vi "Child_2 - Config - RD WR.vi"(8 "Error In":errorcluster, 9 "Create a New Config File?":bool, 11 "In Cluster":T1={"Relative Array of paths"=["API", "Cfg", "Common", "Data", "Data\\Database_Script", "Data\\FW", "Data\\PIC", "Data\\DBC", "Data\\SSL_Certificates", "Debug", "Deployment", "Documentation", "Driver", "SEQ", "SEQ\\PreUUT\\Control", "SEQ\\PreUUT\\Module", "SEQ\\PreUUT\\Scanner", "SEQ\\CodeModule", "Tool", "Util"]}) -> (0 "Error Out":errorcluster, 3 "Out Cluster":T1={"Relative Array of paths"=["API", "Cfg", "Common", "Data", "Data\\Database_Script", "Data\\FW", "Data\\PIC", "Data\\DBC", "Data\\SSL_Certificates", "Debug", "Deployment", "Documentation", "Driver", "SEQ", "SEQ\\PreUUT\\Control", "SEQ\\PreUUT\\Module", "SEQ\\PreUUT\\Scanner", "SEQ\\CodeModule", "Tool", "Util"]})   [LabVIEW 2023, in "Console_Actor.lvlib" / "Console_Class.lvclass"]
uses:
  Console_Class.lvclass
  Child_2 - Config - Data Structure.ctl
  <vilib>/Utility/xml.llb/Write to XML File(string).vi
  <vilib>/Utility/xml.llb/Read From XML File(string).vi
panel:
  out "Stripped File Path":path
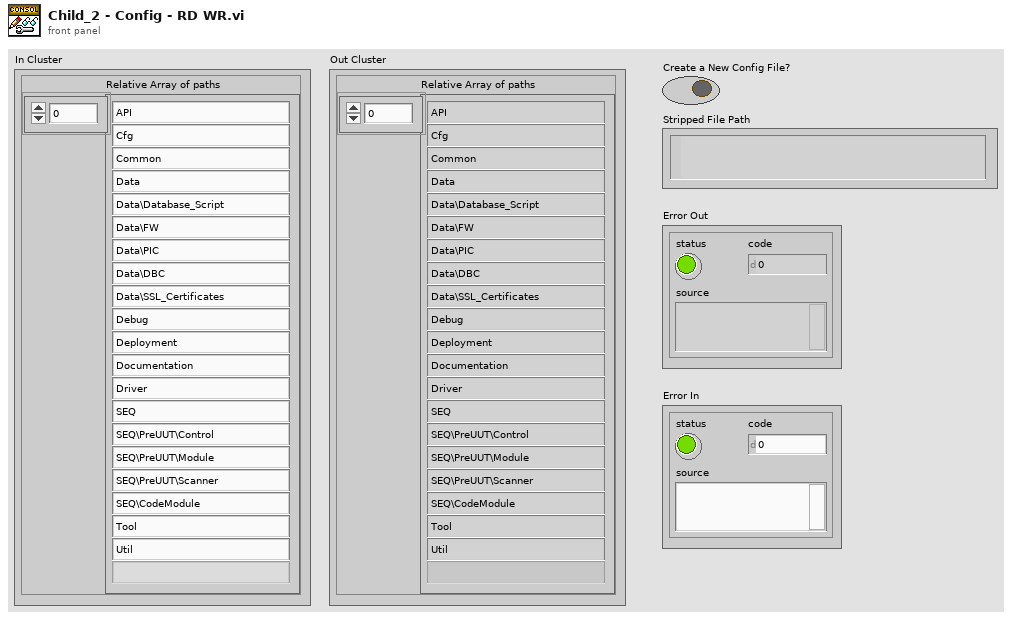
[diagram p1: front panel]
types:
  T1 = typedef "Console_Actor.lvlib/Console_Class.lvclass/Child_2 - Config - Data Structure.ctl" = cluster{"Relative Array of paths":string[]}
  T2 = enum16{"open", "replace", "create", "open or create", "replace or create", "replace or create with confirmation"}
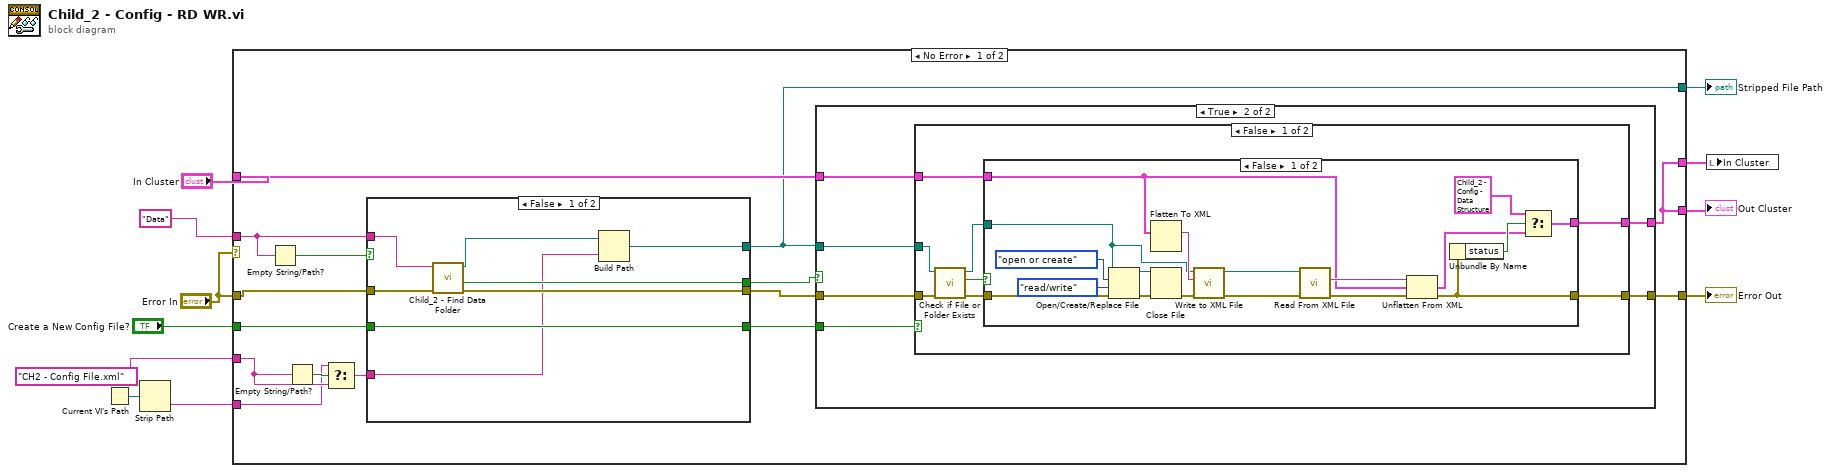
[diagram p0: block diagram]
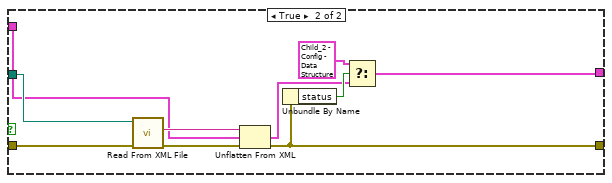
[diagram p3: hidden frame]
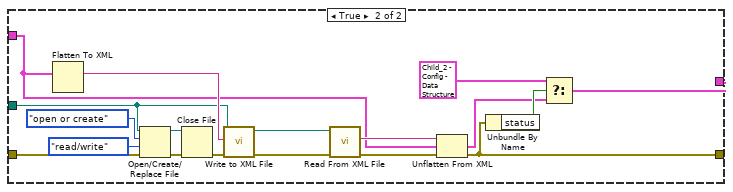
[diagram p4: hidden frame]
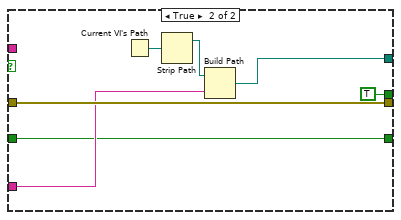
[diagram p5: hidden frame]
diagram:
  n1 = Current VI's Path() -> (path=w4:path)
  n2 = Strip Path(path=w4) -> (name=w3:string)  [unwired: 1 out]
  n3 = case shown="No Error" "Error In" {
    tunnel: "Error In" -> [w24 w103]
    tunnel: "In Cluster" -> [w26 _]
    tunnel: [w25 w103] -> w10
    tunnel: "Create a New Config File?" -> [w22 _]
    tunnel: [w12 _] -> w8
    tunnel: "Data" ("Target Folder to Store XML Config File") -> [w19 _]
    tunnel: "CH2 - Config File.xml" ("XML Config File (if Empty = VI name)") -> [w16 _]
    tunnel: w3 -> [w15 _]
    tunnel: [w13 _] -> w2
    tunnel: [w12 _] -> w1
    frame No Error {
      n4 = Empty String/Path?(string/path=w19) -> (empty?=w20:bool)
      n5 = Empty String/Path?(string/path=w16) -> (empty?=w17:bool)
      n6 = Select(t=w15, s=w17, f=w16) -> (s? t:f=w14:string)
      n7 = case shown="False" w20 {
        tunnel: w24 -> [w95 w99]
        tunnel: [w94 w99] -> w23
        tunnel: w19 -> [w93 _]
        tunnel: [w91 w97] -> w13
        tunnel: w22 -> [w90 w96]
        tunnel: [w90 w96] -> w21
        tunnel: [w89 TRUE ("Pass?")] -> w18
        tunnel: w14 -> [w88 w98]
        frame False {
          n8 = call "Child_2 - Find Data Folder.vi"("Target Folder"=w93, "Error In"=w95) -> ("Target Folder Path"=w92:path, "Pass?"=w89:bool, "Error Out"=w94:errorcluster)  [unwired: 6 in]
          n9 = Build Path(base path=w92, name or relative path=w88) -> (appended path=w91:path)
        }
        frame True {
          n10 = Current VI's Path() -> (path=w100:path)
          n11 = Strip Path(path=w100) -> (stripped path=w101:path)  [unwired: 1 out]
          n12 = Build Path(base path=w101, name or relative path=w98) -> (appended path=w97:path)
        }
      }
      n13 = case shown="True" w18 {
        tunnel: w26 -> [_ w33]
        tunnel: [w27 w32] -> w25
        tunnel: [_ w31] -> w12
        tunnel: w23 -> [w27 w30]
        tunnel: w13 -> [_ w29]
        tunnel: w21 -> [_ w28]
        frame False {
        }
        frame True {
          n14 = case shown="False" w28 {
            tunnel: w30 -> [w41 w75]
            tunnel: [w37 w73] -> w32
            tunnel: [w36 w72] -> w31
            tunnel: w33 -> [w35 w74]
            tunnel: w29 -> [w34 w70]
            frame False {
              n15 = call <vilib>:"Check if File or Folder Exists.vi"("error in (no error)"=w41, "path"=w34) -> ("error out"=w38:errorcluster, "file or folder exists?"=w40:bool, "dup path"=w39:path)  [unwired: 7 in]
              n16 = case shown="False" w40 {
                tunnel: w35 -> [w45 w64]
                tunnel: w39 -> [w51 w66]
                tunnel: w38 -> [w52 w65]
                tunnel: [w44 w63] -> w37
                tunnel: [w50 w61] -> w36
                frame False {
                  n17 = Open/Create/Replace File(file path (use dialog)=w51, error in=w52, operation (0:open)=T2."open or create", access (0:read/write)=enum16{"read/write", "read-only", "write-only"}."read/write") -> (refnum out=w58:refnum<file>, error out=w59:errorcluster)  [unwired: 2 in, 1 out]
                  n18 = Flatten To XML(6:w45) -> (2:w56:string)
                  n19 = Close File(refnum=w58, error in=w59) -> (error out=w57:errorcluster)  [unwired: 1 out]
                  n20 = call-poly <vilib>:"Write to XML File.vi"("error in (no error)"=w57, "XML Input"=w56, "XML File Path"=w51) -> ("error out"=w46:errorcluster, "XML File Path(duplicate)"=w47:path)  [unwired: 6 in, 1 out]
                  n21 = call-poly <vilib>:"Read From XML File.vi"("error in (no error)"=w46, "XML File Path"=w47) -> ("error out"=w48:errorcluster, "XML Elements"=w49:string)  [unwired: 7 in, 1 out]
                  n22 = Unflatten From XML(xml string=w49, type=w45, error in (no error)=w48) -> (value=w43:T1, error out=w44:errorcluster)
                  n23 = Unbundle By Name(w44) -> ("status"=w53:bool)
                  n24 = Select(t=T1 {"Relative Array of paths"=["API", "Cfg", "Common", "Data", "Data\\Database_Script", "Data\\FW", "Data\\PIC", "Data\\DBC", "Data\\SSL_Certificates", "Debug", "Deployment", "Documentation", "Driver", "SEQ", "SEQ\\PreUUT\\Control", "SEQ\\PreUUT\\Module", "SEQ\\PreUUT\\Scanner", "SEQ\\CodeModule", "Tool", "Util"]} ("In Cluster"), s=w53, f=w43) -> (s? t:f=w50:T1)
                }
                frame True {
                  n25 = call-poly <vilib>:"Read From XML File.vi"("error in (no error)"=w65, "XML File Path"=w66) -> ("error out"=w69:errorcluster, "XML Elements"=w68:string)  [unwired: 7 in, 1 out]
                  n26 = Unflatten From XML(xml string=w68, type=w64, error in (no error)=w69) -> (value=w62:T1, error out=w63:errorcluster)
                  n27 = Unbundle By Name(w63) -> ("status"=w67:bool)
                  n28 = Select(t=T1 {"Relative Array of paths"=["API", "Cfg", "Common", "Data", "Data\\Database_Script", "Data\\FW", "Data\\PIC", "Data\\DBC", "Data\\SSL_Certificates", "Debug", "Deployment", "Documentation", "Driver", "SEQ", "SEQ\\PreUUT\\Control", "SEQ\\PreUUT\\Module", "SEQ\\PreUUT\\Scanner", "SEQ\\CodeModule", "Tool", "Util"]} ("In Cluster"), s=w67, f=w62) -> (s? t:f=w61:T1)
                }
              }
            }
            frame True {
              n29 = Flatten To XML(6:w74) -> (2:w84:string)
              n30 = Open/Create/Replace File(file path (use dialog)=w70, error in=w75, operation (0:open)=T2."open or create", access (0:read/write)=enum16{"read/write", "read-only", "write-only"}."read/write") -> (refnum out=w86:refnum<file>, error out=w87:errorcluster)  [unwired: 2 in, 1 out]
              n31 = Close File(refnum=w86, error in=w87) -> (error out=w85:errorcluster)  [unwired: 1 out]
              n32 = call-poly <vilib>:"Write to XML File.vi"("error in (no error)"=w85, "XML Input"=w84, "XML File Path"=w70) -> ("error out"=w77:errorcluster, "XML File Path(duplicate)"=w78:path)  [unwired: 6 in, 1 out]
              n33 = call-poly <vilib>:"Read From XML File.vi"("error in (no error)"=w77, "XML File Path"=w78) -> ("error out"=w79:errorcluster, "XML Elements"=w80:string)  [unwired: 7 in, 1 out]
              n34 = Unflatten From XML(xml string=w80, type=w74, error in (no error)=w79) -> (value=w76:T1, error out=w73:errorcluster)
              n35 = Unbundle By Name(w73) -> ("status"=w81:bool)
              n36 = Select(t=T1 {"Relative Array of paths"=["API", "Cfg", "Common", "Data", "Data\\Database_Script", "Data\\FW", "Data\\PIC", "Data\\DBC", "Data\\SSL_Certificates", "Debug", "Deployment", "Documentation", "Driver", "SEQ", "SEQ\\PreUUT\\Control", "SEQ\\PreUUT\\Module", "SEQ\\PreUUT\\Scanner", "SEQ\\CodeModule", "Tool", "Util"]} ("In Cluster"), s=w81, f=w76) -> (s? t:f=w72:T1)
            }
          }
        }
      }
    }
    frame Error {
    }
  }
  "Error Out" <- w10
  "Out Cluster" <- w8
  "Stripped File Path" <- w2
  n37 = local write "In Cluster"(w1) -> ()
